vi "Day 2.vi"() -> ()   [LabVIEW 2023]
panel:
  out "Oponent":i32
  out "You":i32
  out "array":string[][](array[string])
  in  "input":string="A Z\nA Y\nB X\nB X\nC X\nB X\nA X\nA X\nC X\nA X\nA X\nA Y\nB X\nA Y\nC X\nC X\nA X\nA Y\nC X\nB X\nA X\nB X\nA X\nA X\nB Y\nB Y\nA X\nA X\nA X\nA X\nA X\nA Y\nA X\nB X\nB Y\nA Y\nC Z\nC X\nA X\nA Y\nA X\nA X\nA Y\nA X\nA Y\nA X\nB X\nC X\nA X\nB X\nA X\nC X\nA Y\nB X\nB X\nA X\nA X\nC Y\nB X\nA X\nC X\nB X\nB X\nA X\nA X\nB X\nA Y\nC X\nA Y\nA X\nA X\nA Y\nB X\nA X\nA X\nA X\nB Y\nA X\nA X\nA Y\nA X\nA X\nB Y\nB Y\nB X\nC X\nB Y\nA X\nC X\nC X\nA Y\nA X\nA Z\nB X\nC X\nA Y\nB X\nA X\nA X\nA X\nA Y\nC X\nA X\nA Z\nA X\nA Y\nB Y\nA X\nC X\nB X\nA Y\nB Z\nB X\nC Y\nB X\nB Z\nA Y\nB X\nC X\nC Y\nA X\nA Y\nA X\nB X\nA Y\nB Y\nA X\nC Y\nA Y\nB Y\nA X\nB Y\nB X\nB Y\nA X\nB Y\nA X\nC Z\nA X\nC X\nA Y\nA X\nC X\nA X\nA X\nA X\nC X\nB Z\nA X\nB Y\nB X\nA Y\nA X\nA X\nB Y\nB Y\nA Y\nB X\nA X\nC Y\nA X\nC X\nA X\nA X\nA X\nA X\nA X\nC Z\nC X\nA Z\nC Z\nA X\nA Y\nB X\nC X\nB X\nB Y\nC X\nB X\nA X\nA X\nA X\nA Y\nB X\nB Y\nA X\nC X\nA X\nA X\nA X\nA X\nC Y\nA Z\nC X\nA X\nA Y\nB X\nA Y\nA X\nA Y\nA X\nA X\nA X\nA X\nA Y\nA X\nB X\nA X\nA X\nC Y\nC Y\nA X\nC X\nA X\nA X\nC X\nC X\nB Z\nB X\nB X\nA X\nA Y\nB Y\nA X\nA X\nC X\nC X\nC X\nB X\nC X\nB Y\nA X\nB Y\nB X\nB X\nA X\nB Y\nA Y\nC X\nB X\nC X\nA Y\nB X\nC X\nA X\nC X\nA X\nB Y\nA X\nA X\nB Z\nC X\nB X\nC X\nB X\nA X\nA X\nA X\nA X\nA X\nC X\nC X\nA X\nA Z\nA Y\nA X\nA X\nA X\nA X\nC Y\nC Y\nB Z\nA X\nA X\nB X\nB X\nA Y\nA X\nB Y\nA X\nB Y\nA X\nC Y\nC X\nA Y\nB Y\nC X\nA X\nA X\nA X\nA Y\nA X\nA X\nA X\nB Y\nB X\nC X\nC Y\nA Y\nA Z\nB X\nC X\nB X\nC X\nA X\nB Z\nB Y\nA X\nC X\nA Y\nB X\nB X\nA Y\nA X\nA X\nA Y\nA X\nB X\nA X\nA X\nC Y\nC Y\nA Y\nA Y\nB Y\nB Y\nB Y\nB X\nA X\nA Y\nB Y\nB X\nA Y\nA X\nA Y\nC X\nC X\nB Y\nA Y\nB Y\nA Y\nA X\nB Y\nB X\nC X\nA X\nA X\nA X\nB Y\nB X\nA X\nB Y\nA Y\nA X\nC X\nA X\nB Y\nA X\nA X\nB Y\nA Y\nA X\nC Y\nB Z\nA Y\nC X\nA Y\nA X\nB Y\nA X\nB Y\nB Y\nB X\nB X\nA X\nA X\nC X\nB Y\nB X\nC X\nB Y\nA X\nA X\nA X\nA X\nB Y\nC X\nB X\nA X\nA X\nA Y\nC Y\nA Y\nB X\nA X\nB X\nA X\nA Y\nB Y\nA X\nC X\nC X\nA Y\nB X\nC Y\nA Y\nB X\nA X\nA Y\nC X\nA X\nA X\nB Y\nA Y\nB X\nB Y\nB Y\nA X\nA X\nA X\nB Y\nA Y\nA X\nB X\nA Y\nA Y\nB X\nC Y\nA X\nA Y\nA X\nB X\nA X\nB X\nC Z\nA X\nA X\nB Y\nA X\nA X\nA X\nC Z\nC X\nA Z\nC Y\nB X\nA Y\nB X\nA X\nA Y\nA X\nC X\nA X\nA X\nC Y\nA Z\nC Y\nB Y\nB X\nB X\nA Y\nC X\nB X\nA Z\nA X\nA Z\nC X\nA X\nC Z\nC X\nB Z\nC Y\nB Y\nA X\nB Y\nA X\nA X\nC X\nB X\nA X\nC Z\nB Y\nB Y\nA Y\nB Y\nA X\nA X\nB Y\nA X\nA X\nC Y\nC X\nA X\nC Y\nC X\nB X\nB X\nA X\nB Y\nA Y\nA X\nB Y\nB Y\nB X\nB X\nA X\nB X\nB X\nB Y\nB Y\nC X\nB X\nB X\nA X\nA X\nA X\nA X\nA Y\nC Y\nA X\nA Y\nC Z\nA Y\nC X\nA X\nC Y\nA X\nA X\nA Y\nA Z\nA Y\nA Y\nA X\nA Y\nA Z\nC X\nC Z\nB X\nA X\nA X\nB X\nA X\nA X\nA X\nC X\nA X\nA Y\nA X\nA X\nA Y\nC Z\nC X\nA X\nA X\nA Z\nA X\nC X\nA Y\nC X\nA Y\nC X\nC X\nA X\nA X\nA Y\nB Y\nC X\nC X\nB X\nB Z\nB X\nB X\nA X\nC X\nA Y\nC X\nA Z\nB X\nB Y\nA Y\nA Y\nA X\nA Y\nA X\nA X\nA Y\nA X\nA X\nB Z\nA X\nA X\nA X\nB Y\nB Y\nC Z\nA Y\nA Y\nB Y\nA X\nB X\nC X\nC Y\nC X\nB X\nC X\nA Y\nA X\nA X\nB X\nC X\nB X\nA Y\nB X\nB Z\nA Y\nA X\nA Y\nB X\nB Z\nA X\nA X\nC X\nA X\nA Y\nA X\nB X\nA X\nA X\nA Z\nB X\nB Y\nC Y\nC X\nA Y\nA X\nB Y\nC X\nA X\nC Y\nA X\nA Y\nA Y\nA X\nA X\nC X\nC X\nA Y\nA Y\nC X\nA X\nB X\nC X\nB Y\nC Y\nC X\nB X\nB Y\nC X\nB X\nB Y\nA X\nA X\nB X\nA Y\nA X\nB X\nA X\nC Y\nA X\nB X\nA Y\nC Y\nA X\nA Y\nA Z\nC Z\nA X\nA X\nC X\nA X\nB X\nA X\nC X\nC X\nA Y\nA X\nC Y\nA Y\nA X\nB Y\nA X\nA Y\nA X\nC Z\nC Z\nC X\nA X\nA X\nA X\nA X\nC X\nA X\nC X\nB X\nB X\nA X\nA Y\nB Y\nB X\nB X\nA Y\nA Y\nA X\nA X\nB Y\nB X\nA X\nC X\nB X\nC X\nB Y\nB Z\nB Y\nA X\nA X\nA X\nA X\nA X\nB Y\nA X\nC X\nB Z\nA X\nC Y\nA X\nB X\nC Y\nA X\nA Y\nB X\nA X\nB Y\nB X\nA Y\nC Y\nC X\nA Y\nA X\nA X\nA X\nC X\nB X\nC X\nA Y\nA X\nA Y\nC Z\nC X\nA X\nA Y\nB X\nB X\nB X\nB X\nA X\nB X\nA Z\nB Y\nA X\nA X\nA X\nC Z\nA Y\nA Y\nC X\nC X\nC Y\nB Y\nA Y\nA X\nA X\nC Y\nA X\nC X\nA X\nA X\nC Y\nA Y\nA X\nC X\nA X\nA Y\nC X\nA Y\nA X\nA X\nA X\nB X\nB X\nA X\nB Y\nC Y\nC X\nA Y\nB X\nB X\nB Z\nC X\nB Y\nA Y\nC Z\nB X\nC X\nA X\nA Y\nB Y\nB X\nC Z\nB X\nA X\nC X\nC X\nA X\nA X\nA Y\nB Y\nB X\nA Y\nC Y\nB Y\nB Y\nA X\nA Y\nA X\nB X\nA Y\nA X\nA Y\nA X\nB Z\nB X\nA X\nA Y\nA X\nB Y\nA Y\nA X\nA X\nC X\nA X\nA X\nA X\nA X\nB Y\nB X\nA X\nA X\nC Y\nC X\nA Y\nA X\nB X\nA X\nB X\nB X\nB Y\nA X\nB X\nB Y\nA X\nB X\nC X\nA X\nA X\nC Z\nA X\nB X\nA X\nB X\nB X\nB Y\nA X\nB Y\nC Y\nA X\nC X\nA X\nB X\nB Y\nA X\nC X\nB X\nA X\nC Y\nC X\nB X\nA X\nB X\nA Z\nC Y\nA X\nA X\nB X\nA Y\nB X\nA X\nA Y\nB X\nA X\nC Y\nA X\nC X\nB X\nA X\nC Y\nC X\nA X\nB Y\nB X\nA Y\nB X\nA X\nB X\nA Y\nB X\nA X\nA X\nC X\nA X\nA X\nA X\nA X\nC X\nC X\nB X\nB Y\nB X\nB Z\nA X\nB X\nB Y\nB X\nB X\nA X\nA Z\nA Z\nA X\nB Y\nA X\nB X\nB Y\nA X\nB Y\nB X\nA X\nC X\nC Y\nA X\nA X\nB X\nB X\nB Y\nA X\nC X\nB Y\nA X\nA Z\nA X\nC Y\nA Y\nB X\nC X\nC X\nA X\nB X\nC X\nA Z\nA X\nA X\nB Y\nC X\nA X\nA Y\nC Z\nB X\nA Y\nA X\nA Z\nC Y\nA X\nC X\nA X\nC Y\nB X\nA X\nA X\nB Y\nA X\nB X\nB X\nB X\nC X\nC X\nA X\nC Z\nA X\nC Y\nA X\nC Y\nA Y\nB Y\nB X\nB Y\nB X\nC Y\nB Y\nB Y\nB X\nB Y\nA Y\nA Y\nC Z\nA X\nA X\nA X\nA Z\nB X\nB Y\nB X\nB Y\nA X\nC X\nB X\nA X\nC Y\nB X\nC X\nC Y\nB Y\nA X\nB Y\nB X\nC X\nB X\nC X\nB X\nA X\nC X\nB Z\nB Z\nC X\nA Y\nB X\nA Y\nA X\nB X\nC Y\nC X\nA Y\nC Y\nB Z\nB Y\nB Y\nB Y\nB Z\nB Y\nA X\nA X\nA Y\nB Y\nB Y\nA X\nA Z\nC X\nA X\nA Y\nC X\nA Y\nA X\nB X\nA X\nA X\nC X\nA X\nA X\nC Y\nB Y\nA Y\nA X\nA X\nB Y\nA X\nB X\nA X\nA X\nB X\nB X\nA X\nB Y\nA X\nA Y\nB Y\nA Y\nA X\nC X\nA Y\nA X\nC X\nA X\nA X\nB X\nC Y\nC Y\nB X\nB Z\nA X\nA Y\nA X\nA X\nC Z\nA X\nB X\nA Z\nA X\nA X\nA X\nA X\nA X\nA X\nC X\nB X\nB X\nC X\nA X\nA X\nA X\nA X\nA X\nA X\nB X\nA X\nC X\nA Y\nA X\nA X\nA X\nA X\nB X\nB Y\nA Y\nA X\nA X\nC X\nC X\nA X\nA X\nC X\nA X\nA X\nA X\nA X\nA X\nA X\nC X\nA X\nA X\nA X\nA X\nB X\nA X\nA X\nB Y\nC Y\nA X\nA Y\nC Y\nA X\nB X\nB X\nA X\nA X\nA X\nB X\nA X\nA X\nA X\nA Y\nA X\nB Y\nA Y\nA X\nA Y\nA X\nC X\nA X\nC Y\nB X\nB X\nA X\nA X\nA X\nA X\nA X\nC Y\nA Z\nA X\nB X\nB X\nA X\nA X\nC Z\nA X\nB Z\nB Y\nC Y\nA X\nA X\nC X\nB X\nB X\nB X\nC X\nA X\nA Y\nB Y\nC X\nA X\nB Y\nA X\nC Z\nB X\nA Y\nA X\nA X\nC Y\nA X\nA X\nC X\nA X\nB X\nB Y\nB Y\nB X\nA X\nA Y\nC X\nA X\nA X\nA X\nB X\nC X\nB Y\nA X\nA X\nA Y\nA X\nA X\nB X\nC X\nC X\nA Y\nB X\nA X\nA X\nA X\nB Y\nA X\nB X\nA X\nA X\nA X\nA Y\nA X\nA Z\nC X\nB Y\nB X\nA X\nB X\nC X\nA X\nA X\nB X\nA X\nA X\nA X\nA X\nB X\nA X\nC X\nA Y\nB X\nC X\nA X\nB X\nA X\nB Y\nA X\nC Y\nA X\nC Y\nC X\nB Y\nA Y\nA X\nA X\nB X\nA X\nC X\nA X\nA Z\nB X\nA X\nA X\nA Y\nA X\nA X\nC X\nB Y\nC Z\nA X\nA Y\nB X\nB X\nA X\nB Y\nC X\nA X\nB X\nA Y\nB X\nA X\nA Y\nA X\nA X\nC Y\nB X\nA Y\nC X\nC X\nA Y\nA Y\nA X\nB Z\nA Y\nC X\nC X\nC Y\nA Y\nB X\nB Z\nA X\nB Y\nA X\nA X\nB X\nA Y\nC X\nC Y\nA X\nB Y\nA Y\nA X\nB Z\nB Y\nA X\nB X\nA X\nA X\nB Y\nA Y\nA X\nA X\nA X\nA Y\nA X\nA X\nC X\nA X\nA X\nC X\nA X\nA X\nC Z\nB X\nA Y\nA X\nB Y\nB X\nA X\nA X\nA X\nC Y\nC Y\nB Y\nA X\nC X\nC X\nB X\nA X\nA X\nA X\nA Y\nA X\nA X\nB Z\nC X\nA X\nA X\nA X\nB Y\nB X\nC X\nB X\nA X\nB X\nA X\nC X\nA X\nC X\nA X\nC X\nB Y\nB X\nA X\nA X\nB Y\nB X\nB X\nA X\nB X\nC Y\nA X\nA Y\nA Y\nA Y\nA Z\nB Y\nA X\nA X\nA X\nA X\nA Z\nA X\nA X\nA X\nB Z\nB Y\nC Y\nA X\nA X\nB X\nC X\nA Y\nA X\nB X\nA X\nA X\nB X\nB Y\nA X\nB X\nC X\nB X\nA X\nA X\nA X\nA X\nB X\nB X\nC Y\nB X\nB X\nA X\nB X\nA X\nB Y\nB X\nA X\nA X\nA Y\nB X\nA X\nB Y\nA Y\nB Y\nB X\nA Z\nA X\nB Y\nA X\nB X\nA X\nA X\nA X\nB Y\nB X\nA X\nC Z\nA Y\nA Y\nC X\nB Z\nB X\nC Z\nB X\nB X\nA X\nA X\nB Y\nC X\nA X\nA Z\nB X\nA X\nA X\nB Y\nA X\nA X\nA X\nB Y\nA X\nC Y\nA X\nC Y\nA X\nC Y\nB X\nA Y\nA X\nB X\nA X\nB Y\nA X\nB X\nB X\nA Z\nA X\nC Y\nB Y\nA X\nA X\nC X\nB Y\nC Y\nC X\nA Y\nB Y\nA Y\nA Y\nB X\nA X\nA X\nA X\nA X\nA Y\nA X\nA X\nA X\nB Y\nA X\nA Y\nC X\nA X\nB X\nA X\nA X\nA X\nC Z\nA X\nA Y\nA X\nC Z\nB Y\nB X\nA X\nA Z\nA X\nA X\nA Y\nA X\nA X\nA X\nB Y\nA X\nB X\nA X\nA X\nA X\nA X\nB X\nB Z\nC X\nC X\nC X\nB Y\nA X\nB Y\nB X\nA Y\nB X\nB X\nA X\nC Y\nB X\nA X\nA X\nA X\nA X\nA X\nA X\nB Y\nC Y\nB X\nC Y\nB Y\nC X\nA Y\nC X\nB X\nC X\nB X\nA X\nA X\nB Y\nA X\nC X\nA Y\nC X\nC X\nB Y\nA X\nC X\nC X\nB Z\nA X\nC X\nA Y\nB Y\nA X\nA Y\nA X\nB X\nA X\nA X\nB Y\nA Z\nA X\nB Y\nB X\nA X\nA Y\nB X\nB X\nA X\nA X\nA Y\nA X\nC X\nA X\nB X\nC X\nC X\nC Y\nA X\nB X\nB Y\nA X\nC X\nA X\nB Y\nA X\nB X\nB Z\nA X\nA X\nA X\nB X\nC X\nC X\nB X\nA Y\nA X\nA Y\nA X\nA X\nA X\nA X\nC Y\nB X\nA X\nA X\nA X\nB Y\nA X\nB X\nB Y\nA Z\nA Y\nA X\nA Y\nA X\nA Y\nB Z\nA X\nB Y\nB Z\nB X\nA X\nC X\nC Y\nA X\nA X\nA X\nB X\nA Y\nC X\nA X\nB Y\nA Y\nB X\nB X\nA X\nA Y\nB X\nA Y\nC X\nA X\nC X\nA X\nC X\nA X\nA X\nC X\nA X\nA X\nA Y\nB X\nC X\nB Y\nA Y\nA X\nA X\nA X\nA Z\nB Y\nA X\nA X\nB Y\nA Y\nB Y\nA X\nB Y\nB X\nA X\nA X\nA X\nB X\nB Y\nA X\nC Z\nB Z\nA X\nA X\nA X\nB X\nB Y\nA X\nB Z\nA X\nA Y\nA Y\nA Y\nC X\nB Y\nA X\nA X\nC Y\nB X\nA Y\nA X\nA X\nB Y\nC X\nC X\nC X\nA X\nA X\nA X\nB Z\nA X\nC X\nA X\nA X\nB X\nB X\nA X\nC Y\nA X\nB X\nC X\nB Y\nA X\nB Y\nC X\nA X\nC X\nB Y\nA X\nA Y\nC X\nC Z\nA X\nC X\nA X\nA X\nC X\nA Y\nC X\nB Y\nA X\nC Z\nA X\nB X\nB Y\nA Y\nA X\nA X\nA X\nA X\nA Y\nA Y\nB X\nC X\nA Y\nA X\nC X\nB X\nB Y\nC X\nB X\nA X\nB X\nA X\nC Y\nA X\nA X\nA X\nA X\nC X\nA X\nB X\nA X\nB X\nA X\nA Y\nC X\nC Y\nC X\nA Z\nB X\nA Z\nA X\nB Y\nA Y\nB X\nA X\nB Y\nA Y\nA X\nB Y\nA X\nB X\nA X\nA X\nA X\nA X\nB Y\nA Y\nA X\nA X\nB X\nB Z\nA Y\nA Y\nC Y\nC Y\nA X\nC X\nA X\nB Y\nB X\nB Y\nB X\nC X\nB X\nC X\nA X\nB Y\nA X\nB X\nA X\nB X\nC Y\nB X\nA X\nA Y\nA X\nB Y\nC X\nC X\nA X\nB Z\nA X\nA X\nB Y\nA X\nA X\nB X\nA Y\nC X\nA X\nC Y\nA Y\nC X\nA Y\nA X\nA X\nA X\nA Y\nB X\nB X\nA Y\nC X\nB Y\nA Y\nB X\nB X\nB X\nB X\nA X\nB X\nB X\nA X\nC X\nA X\nC X\nC X\nA X\nC X\nB X\nA Y\nA Z\nA X\nA X\nA X\nA Y\nA X\nA X\nC Z\nA X\nB X\nC X\nA X\nB X\nC X\nC X\nA X\nB Y\nA X\nA X\nA X\nA Y\nB Y\nB Y\nA X\nB X\nA X\nC X\nA X\nB Y\nC Y\nC X\nC X\nB X\nB X\nC X\nA Y\nB X\nA X\nA X\nA X\nA X\nA Y\nB X\nB X\nC Y\nC Y\nB Y\nB X\nA X\nC Y\nA X\nC Z\nC X\nA X\nB Z\nA X\nA Z\nC X\nB Y\nA X\nA Y\nA X\nB X\nA Y\nC X\nC Y\nB X\nB X\nB Y\nB Y\nC X\nB Y\nB Y\nB X\nC X\nC X\nA X\nA X\nA Y\nA X\nA Y\nB X\nA X\nB Y\nB X\nA X\nA X\nA Y\nB X\nB X\nA X\nB X\nC Y\nA Y\nB Y\nC Y\nB Y\nA X\nB Y\nB X\nB Z\nA Y\nA Y\nC Y\nB X\nA X\nA X\nB Y\nA X\nA X\nB X\nA X\nA X\nA X\nB X\nB X\nB Y\nA X\nC X\nA X\nB X\nA X\nA X\nA Y\nB X\nB X\nB X\nC X\nB Y\nC Z\nA X\nC X\nA X\nB X\nA X\nA Y\nB Y\nA Z\nA X\nC X\nA Y\nA X\nA X\nA X\nA X\nA Y\nA X\nC X\nA X\nC Y\nB X\nA X\nA X\nA X\nA X\nA X\nC X\nA X\nB X\nB Y\nB Y\nB X\nC Z\nC X\nB X\nC Y\nA X\nA X\nA X\nA X\nA X\nC X\nA X\nB X\nC X\nC X\nA X\nA X\nB X\nA X\nA X\nA X\nB X\nA X\nC X\nA X\nA Y\nA X\nB Y\nA X\nB X\nA Y\nC X\nB X\nC Y\nC Y\nB X\nA X\nB X\nC X\nA X\nC X\nA X\nC X\nB X\nB X\nC X\nC X\nB X\nB X\nC Y\nB X\nA X\nB X\nB X\nB Y\nA Y\nB X\nA X\nC Y\nA Y\nC Y\nA X\nB Y\nA X\nA X\nA X\nB Y\nB X\nA Y\nA X\nA X\nA Y\nB X\nB Y\nA Y\nB X\nC X\nC Z\nB X\nA Y\nA X\nC X\nA X\nC X\nB Z\nC X\nA Y\nA X\nC X\nB Y\nA Z\nB Y\nA X\nA X\nA Y\nC X\nA Z\nA X\nB Y\nA X\nB X\nA Y\nA Y\nA X\nA X\nA X\nC Y\nB X\nA X\nB X\nB Y\nB Y\nA X\nA X\nA Y\nA X\nC X\nB X\nC X\nB X\nB X\nC Y\nA Y\nB X\nA X\nA X\nA X\nC X\nC X\nA X\nB X\nA X\nA X\nA Z\nA X\nC X\nB X\nA X\nC Y\nA Y\nC Y\nB Y\nB Y\nB Z\nA X\nC X\nA X\nB Y\nB Y\nA X\nB Y\nA X\nB Y\nB X\nB X\nC X\nB Y\nB X\nA X\nA Y\nB X\nA X\nB Z\nA Y\nB X\nB X\nA Y\nC Y\nB X\nB Y\nA X\nB X\nA Y\nA Y\nB X\nB Y\nB X\nA X\nC X\nA X\nA X\nA X\nB Y\nA Y\nB X\nC X\nC Z\nA X\nB Y\nA Y\nA X\nB X\nA X\nA Y\nA X\nA Y\nA X\nA X\nA X\nC X\nA Y\nC Y\nA X\nA X\nC Z\nB X\nA Y\nB X\nB X\nB X\nB X\nB X\nA X\nA X\nB X\nB Y\nA X\nC Y\nC X\nA X\nA X\nA X\nA X\nA X\nA X\nA X\nA Y\nB Y\nA X\nA X\nA Z\nC Y\nC Y\nB X\nC Z\nA X\nA X\nA X\nB Z\nB Y\nA X\nA X\nA X\nB X\nA X\nC X\nC X\nC X\nB X\nA X\nA X\nC Z\nB Z\nC Y\nA X\nA X\nA X\nC Z\nA X\nA X\nC X\nC X\nA X\nC Y\nA X\nA Y\nA X\nA X\nA Z\nC X\nC X\nA Y\nB X\nB X\nA Y\nA X\nB X\nC Y\nA X\nA Y\nB Z\nA X\nC Y\nA X\nB Y\nA X\nA Y\nA X\nC Z\nA X\nB X\nA X\nB Y\nA X\nA X\nA X\nA X\nA X\nB Y\nC X\nA X\nB X\nA X\nA Y\nA Z\nA X\nA X\nB Y\nB X\nC X\nA X\nA X\nB X\nB Y\nB Y\nA Y\nB Z\nB Y\nA X\nA X\nA X\nA X\nB X\nC Y\nA X\nA X\nA X\nA X\nA X\nA X\nA X\nA X\nB Y\nA X\nB X\nC X\nC X\nC X\nC X\nA X\nB Y\nA X\nB X\nB X\nA X\nA X\nC Z\nA X\nB X\nB X\nC X\nA X\nB X\nB X\nB X\nB X\nB Y\nA X\nB X\nA Y\nA X\nA Y\nB Y\nA X\nC Y\nB X\nA X\nA X\nA X\nA Z\nA Y\nA X\nC X\nC X\nB X\nA X\nA X\nB X\nA X\nA Y\nC Z\nA Y\nB X\nB Y\nA X\nC Y\nB Z\n"
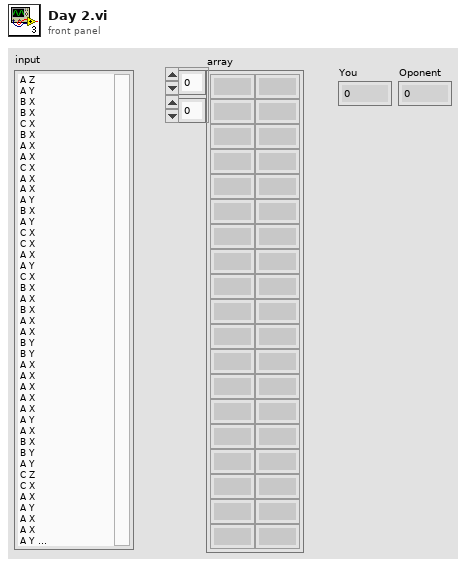
[diagram p1: front panel]
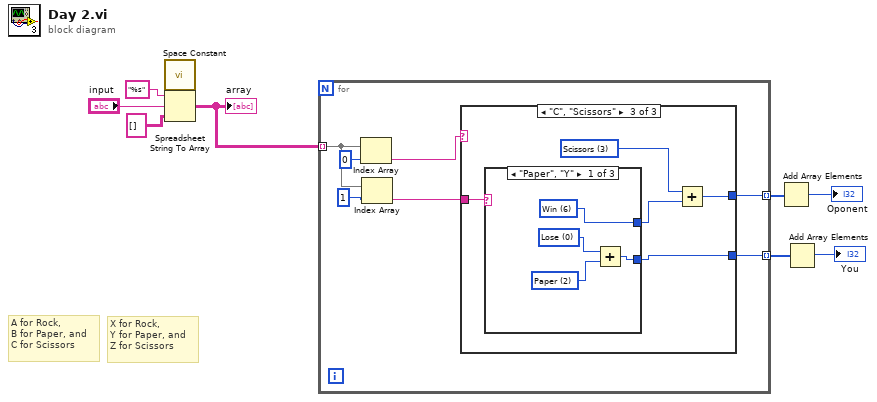
[diagram p0: block diagram]
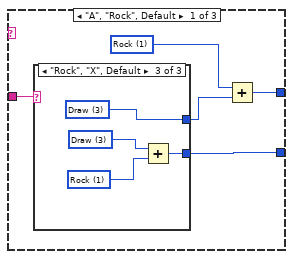
[diagram p2: hidden frame]
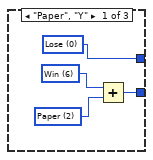
[diagram p3: hidden frame]
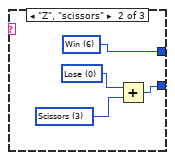
[diagram p4: hidden frame]
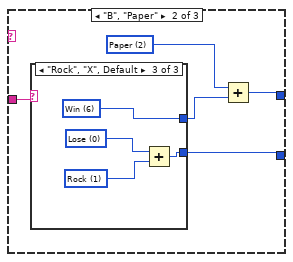
[diagram p5: hidden frame]
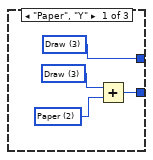
[diagram p6: hidden frame]
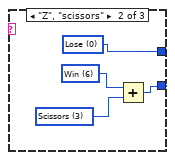
[diagram p7: hidden frame]
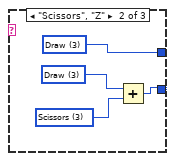
[diagram p8: hidden frame]
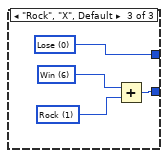
[diagram p9: hidden frame]
diagram:
  # "A for Rock, \nB for Paper, and \nC for Scissors"
  # "X for Rock, \nY for Paper, and \nZ for Scissors"
  n1 = call <vilib>:"Space Constant.vi"() -> ("String"=w7:string)
  n2 = Spreadsheet String To Array(delimiter (Tab)=w7, format string="%s", spreadsheet string="input", array type (2D Dbl)=string[][] [] ("decimal integer string")) -> (array=w5:string[][])
  "array" <- w5
  n3 = for {
    tunnel: w5 -> [w16] mode=indexing
    tunnel: [w11] -> w2 mode=indexing
    tunnel: [w10] -> w1 mode=indexing
    n4 = Index Array(array=w16, index=0) -> (element=w13:string)
    n5 = Index Array(array=w16, index=1) -> (element=w12:string)
    n6 = case shown="\"C\", \"Scissors\"" w13 {
      tunnel: w12 -> [w17 w34 w51]
      tunnel: [w19 w36 w53] -> w11
      tunnel: [w18 w35 w52] -> w10
      frame "A", "Rock", Default {
        w21 = u16 1 items=["Rock"=1, "Paper"=2, "Scissors"=3]
        n7 = case shown="\"Rock\", \"X\", Default" w17 {
          tunnel: [w22 w26 w30] -> w20
          tunnel: [w23 w27 w31] -> w18
          frame "Paper", "Y" {
            w25 = u16 6 items=["Win"=6, "Draw"=3, "Lose"=0]
            w22 = u16 0 items=["Win"=6, "Draw"=3, "Lose"=0]
            w24 = u16 2 items=["Rock"=1, "Paper"=2, "Scissors"=3]
            n8 = Add(x=w25, y=w24) -> (x+y=w23:u16)
          }
          frame "Z", "scissors" {
            w29 = u16 0 items=["Win"=6, "Draw"=3, "Lose"=0]
            w26 = u16 6 items=["Win"=6, "Draw"=3, "Lose"=0]
            w28 = u16 3 items=["Rock"=1, "Paper"=2, "Scissors"=3]
            n9 = Add(x=w29, y=w28) -> (x+y=w27:u16)
          }
          frame "Rock", "X", Default {
            w33 = u16 3 items=["Win"=6, "Draw"=3, "Lose"=0]
            w30 = u16 3 items=["Win"=6, "Draw"=3, "Lose"=0]
            w32 = u16 1 items=["Rock"=1, "Paper"=2, "Scissors"=3]
            n10 = Add(x=w33, y=w32) -> (x+y=w31:u16)
          }
        }
        n11 = Add(x=w21, y=w20) -> (x+y=w19:u16)
      }
      frame "B", "Paper" {
        w38 = u16 2 items=["Rock"=1, "Paper"=2, "Scissors"=3]
        n12 = case shown="\"Rock\", \"X\", Default" w34 {
          tunnel: [w39 w43 w47] -> w37
          tunnel: [w40 w44 w48] -> w35
          frame "Paper", "Y" {
            w42 = u16 3 items=["Win"=6, "Draw"=3, "Lose"=0]
            w39 = u16 3 items=["Win"=6, "Draw"=3, "Lose"=0]
            w41 = u16 2 items=["Rock"=1, "Paper"=2, "Scissors"=3]
            n13 = Add(x=w42, y=w41) -> (x+y=w40:u16)
          }
          frame "Z", "scissors" {
            w46 = u16 6 items=["Win"=6, "Draw"=3, "Lose"=0]
            w43 = u16 0 items=["Win"=6, "Draw"=3, "Lose"=0]
            w45 = u16 3 items=["Rock"=1, "Paper"=2, "Scissors"=3]
            n14 = Add(x=w46, y=w45) -> (x+y=w44:u16)
          }
          frame "Rock", "X", Default {
            w50 = u16 0 items=["Win"=6, "Draw"=3, "Lose"=0]
            w47 = u16 6 items=["Win"=6, "Draw"=3, "Lose"=0]
            w49 = u16 1 items=["Rock"=1, "Paper"=2, "Scissors"=3]
            n15 = Add(x=w50, y=w49) -> (x+y=w48:u16)
          }
        }
        n16 = Add(x=w38, y=w37) -> (x+y=w36:u16)
      }
      frame "C", "Scissors" {
        w55 = u16 3 items=["Rock"=1, "Paper"=2, "Scissors"=3]
        n17 = case shown="\"Paper\", \"Y\"" w51 {
          tunnel: [w56 w60 w64] -> w54
          tunnel: [w57 w61 w65] -> w52
          frame "Paper", "Y" {
            w59 = u16 0 items=["Win"=6, "Draw"=3, "Lose"=0]
            w56 = u16 6 items=["Win"=6, "Draw"=3, "Lose"=0]
            w58 = u16 2 items=["Rock"=1, "Paper"=2, "Scissors"=3]
            n18 = Add(x=w59, y=w58) -> (x+y=w57:u16)
          }
          frame "Scissors", "Z" {
            w63 = u16 3 items=["Win"=6, "Draw"=3, "Lose"=0]
            w60 = u16 3 items=["Win"=6, "Draw"=3, "Lose"=0]
            w62 = u16 3 items=["Rock"=1, "Paper"=2, "Scissors"=3]
            n19 = Add(x=w63, y=w62) -> (x+y=w61:u16)
          }
          frame "Rock", "X", Default {
            w67 = u16 6 items=["Win"=6, "Draw"=3, "Lose"=0]
            w64 = u16 0 items=["Win"=6, "Draw"=3, "Lose"=0]
            w66 = u16 1 items=["Rock"=1, "Paper"=2, "Scissors"=3]
            n20 = Add(x=w67, y=w66) -> (x+y=w65:u16)
          }
        }
        n21 = Add(x=w55, y=w54) -> (x+y=w53:u16)
      }
    }
  }
  n22 = Add Array Elements(numeric array=w2) -> (sum=→"Oponent":u16)
  n23 = Add Array Elements(numeric array=w1) -> (sum=→"You":u16)
